vi "PictureAdjust.vi"(10 "image data":T1, 11 "Picture in":refnum<vi>) -> (3 "Numeric":dbl)   [LabVIEW 2020]
uses:
  <vilib>/picture/picture.llb/imagedata.ctl
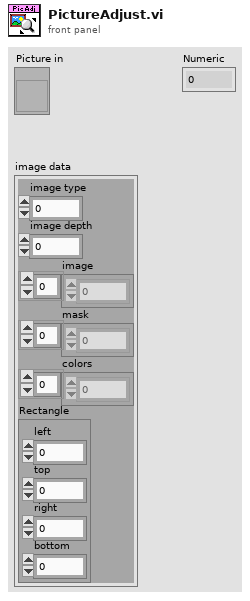
[diagram p1: front panel]
types:
  T1 = typedef "imagedata.ctl" = cluster{"image type":i32, "image depth":i32, "image":u8[], "mask":u8[], "colors":u32[], "Rectangle":cluster{"left":i16, "top":i16, "right":i16, "bottom":i16}}
  T2 = typedef "LVBoundsTypeDef.ctl" = cluster{"Width":u32, "Height":u32}
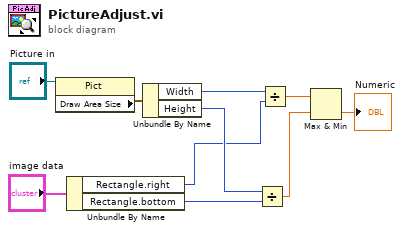
[diagram p0: block diagram]
diagram:
  n1 = property on="Property Node" class="Pict"(reference="Picture in") -> ("Draw Area Size"=w6:T2)  [unwired: 1 in, 2 out]
  n2 = Unbundle By Name("image data") -> ("Rectangle.right"=w2:i16, "Rectangle.bottom"=w8:i16)
  n3 = Unbundle By Name(w6) -> ("Width"=w1:u32, "Height"=w7:u32)
  n4 = Divide(x=w7, y=w8) -> (x/y=w9:dbl)
  n5 = Divide(x=w1, y=w2) -> (x/y=w3:dbl)
  n6 = Max & Min(x=w3, y=w9) -> (min(x,y)=→"Numeric":dbl)  [unwired: 1 out]
